vi "Get All.vi"(8 "error in (no error)":errorcluster, 11 "UserPwd DB in":refnum<class "UserPwd DB.lvclass">) -> (0 "error out":errorcluster, 1 "Access Levels":T1[](array[typedef]), 2 "Usernames":string[](array[string]), 3 "UserPwd DB out":refnum<class "UserPwd DB.lvclass">, 4 "2D Array of Permissions":bool[][](array[boolean]))   [LabVIEW 2016, in "UserPwd DB.lvlib" / "UserPwd DB.lvclass"]
uses:
  <userlib>/Common Components/UserPwd DB/UserPwd DB/UserPwd DB.lvclass
  <userlib>/Common Components/UserPwd DB/UserPwd DB/Access Level.ctl
  <userlib>/Common Components/UserPwd DB/UserPwd DB/UserPwd DB.lvclass/UserPwd DB.ctl
  <userlib>/Common Components/UserPwd DB/UserPwd DB/Data saved.ctl
  <vilib>/addons/_JKI.lib/Serialization/JSON/JKI JSON Serialization.lvlib
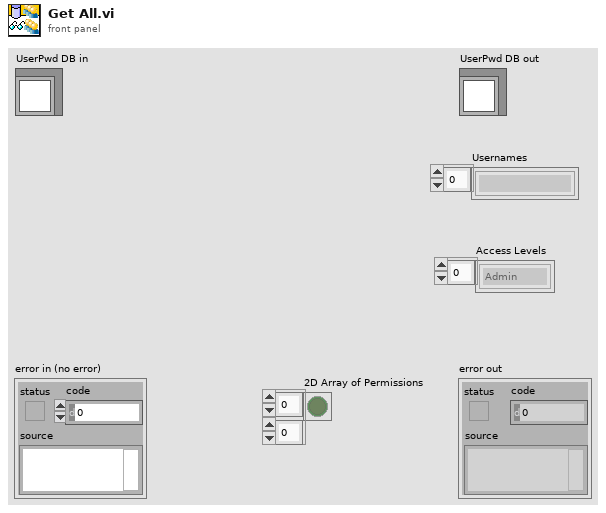
[diagram p1: front panel]
types:
  T1 = typedef "UserPwd DB.lvlib/UserPwd DB.lvclass/Access Level.ctl" = enum16{"Admin", "User lv1", "User lv2", "User lv3", "User lv4", "User lv5", "User lv6", "User lv7", "User lv8", "User lv9", "Guest"}
  T2 = typedef "UserPwd DB.lvlib/UserPwd DB.lvclass/Data saved.ctl" = cluster{"Encrypted Password":string, "Access":T1, "Permission":u32}
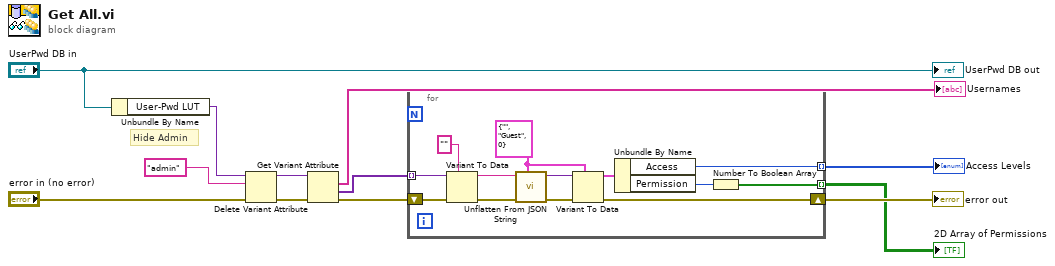
[diagram p0: block diagram]
diagram:
  # "Hide Admin"
  n1 = Unbundle By Name("UserPwd DB in") -> ("User-Pwd LUT"=w4:variant)
  n2 = Delete Variant Attribute(4:"error in (no error)", 6:"admin" ("name (all attributes)"), 7:w4) -> (0:w5:errorcluster, 3:w3:variant)  [unwired: 1 out]
  n3 = Get Variant Attribute(Variant=w3, error in=w5) -> (names=→"Usernames":string[], values=w7:variant[], error out=w9:errorcluster)  [unwired: 2 in, 1 out]
  n4 = for {
    shift-right: [w18] -> w8
    shift-left: w9 -> [w25]
    tunnel: w7 -> [w23] mode=indexing
    tunnel: [w22] -> w6 mode=indexing
    tunnel: [w13] -> w1 mode=indexing
    w16 = T2 {"Encrypted Password"="", "Access"=enum."Guest", "Permission"=0} ("Data")
    n5 = Variant To Data(error in=w25, type="" ("Password"), Variant=w23) -> (data=w19:string, error out=w24:errorcluster)
    n6 = call <vilib>:"Unflatten From JSON String.vi"("Type and Defaults"=w16, "error in (no error)"=w24, "JSON String"=w19) -> ("error out"=w20:errorcluster, "Variant"=w17:variant)  [unwired: 7 in]
    n7 = Variant To Data(error in=w20, type=w16, Variant=w17) -> (data=w15:T2, error out=w18:errorcluster)
    n8 = Unbundle By Name(w15) -> ("Access"=w22:T1, "Permission"=w14:u32)
    n9 = Number To Boolean Array(number=w14) -> (Boolean array=w13:bool[])
  }
  "error out" <- w8
  "Access Levels" <- w6
  "2D Array of Permissions" <- w1
  "UserPwd DB out" <- "UserPwd DB in"
